vi "InitCmdComms.vi"(8 "error in (no error)":errorcluster, 11 "C37.118 PMU in":refnum<class "C37.118 PMU.lvclass">) -> (0 "error out":errorcluster, 3 "C37.118 PMU out":refnum<class "C37.118 PMU.lvclass">)   [LabVIEW 2014, in "SensorPlugins.lvlib" / "C37.118 PMU.lvclass"]
uses:
  C37.118 PMU.lvclass
  C37.118 PMU.lvclass/C37.118 PMU.ctl
  <userlib>/NIST/Socket Class/Classes/Socket.Base/Socket.Base.lvclass/Socket.Base.ctl
  <userlib>/NIST/Socket Class/Classes/Socket.Base/Socket.Base.lvclass
  <userlib>/NIST/Socket Class/Classes/Socket.TCP/Socket.TCP.lvclass
  <userlib>/NIST/Socket Class/Classes/Socket.UDP/Socket.UDP.lvclass
  Accessors/Write CmdSocket.vi
  Accessors/Read CmdSocket.vi
  Accessors/Read PMUComms.vi
  <userlib>/NIST/Socket Class/Classes/Socket.Base/Accessors/Read initialized.vi
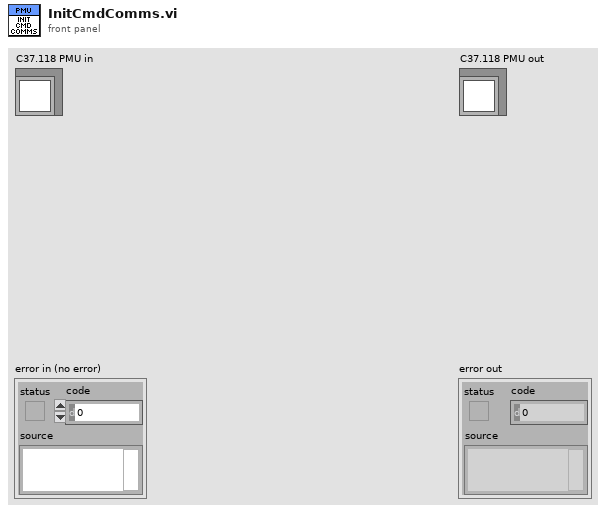
[diagram p1: front panel]
types:
  T1 = typedef "SensorPlugins.lvlib/C37.118 PMU.lvclass/PMUComms.ctl" = cluster{"PMU IP Address":string, "CMD Comms Type":T2, "Data Comms Type":T2, "CMD Port":u16, "Data Port":u16, "PMU ID":u16}
  T2 = typedef "SensorPlugins.lvlib/C37.118 PMU.lvclass/eCommsType.ctl" = enum16{"TCP", "UDP", "USB", "GPIB"}
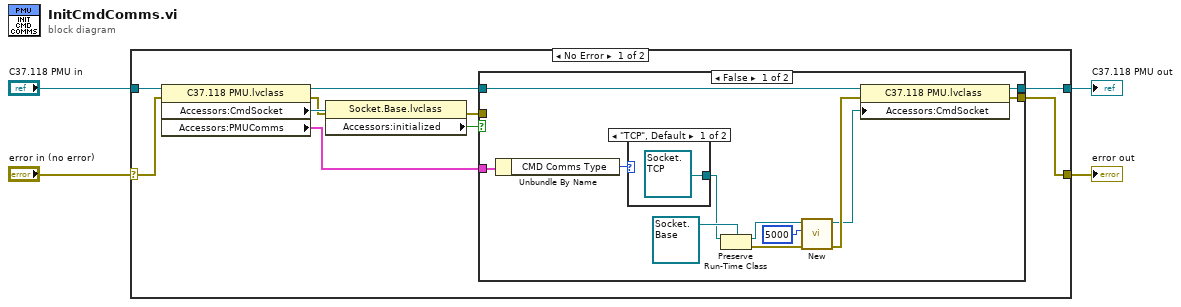
[diagram p0: block diagram]
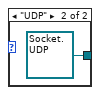
[diagram p2: hidden frame]
diagram:
  n1 = case shown="No Error" "error in (no error)" {
    selector: "error in (no error)" -> [w13 w32]
    tunnel: [w11 w32] -> w3
    tunnel: [w10 w31] -> w1
    tunnel: "C37.118 PMU in" -> [w14 w31]
    frame No Error {
      n2 = property class="C37.118 PMU.lvclass"(reference=w14, error in=w13) -> (reference out=w12:refnum<class "C37.118 PMU.lvclass">, error out=w7:errorcluster, "Accessors:CmdSocket"=w8:refnum<class "Socket.Base.lvclass">, "Accessors:PMUComms"=w9:T1)
      n3 = property class="Socket.Base.lvclass"(reference=w8, error in=w7) -> (error out=w5:errorcluster, "Accessors:initialized"=w6:bool)  [unwired: 1 out]
      n4 = case shown="False" w6 {
        tunnel: w12 -> [w26 w30]
        tunnel: [w25 w29] -> w11
        tunnel: [w24 w30] -> w10
        tunnel: w9 -> [w21 _]
        tunnel: w5 -> [_ w29]
        frame False {
          n5 = Unbundle By Name(w21) -> ("CMD Comms Type"=w20:T2)
          n6 = case shown="\"TCP\", Default" w20 {
            tunnel: [refnum<class "Socket.TCP.lvclass"> refnum ("Socket.TCP in") refnum<class "Socket.UDP.lvclass"> refnum ("Socket.UDP in")] -> w15
            frame "TCP", Default {
            }
            frame "UDP" {
            }
          }
          n7 = Preserve Run-Time Class(object in=w15, 2:refnum<class "Socket.Base.lvclass"> refnum ("Socket.Base in")) -> (object out=w19:refnum<class "Socket.Base.lvclass">, error out=w18:errorcluster)  [unwired: 1 in]
          n8 = call-dynamic "New.vi"("error in (no error)"=w18, "timeout"=5000, "Socket.Base in"=w19) -> ("error out"=w23:errorcluster, "Socket.Base out"=w22:refnum<class "Socket.Base.lvclass">)  [unwired: 7 in]
          n9 = property class="C37.118 PMU.lvclass"(reference=w26, error in=w23, "Accessors:CmdSocket"=w22) -> (reference out=w24:refnum<class "C37.118 PMU.lvclass">, error out=w25:errorcluster)
        }
        frame True {
        }
      }
    }
    frame Error {
    }
  }
  "error out" <- w3
  "C37.118 PMU out" <- w1
